vi "simplePID.vi"(8 "PID Gains":cluster{"Kp":dbl, "Kd":dbl, "Ki":dbl}, 10 "Position":dbl, 11 "Reference":dbl) -> (3 "control":dbl)   [LabVIEW 2010, in "kevLib2011.lvlib"]
uses:
  kevLib2011.lvlib
panel:
  # "Not Tested yet"
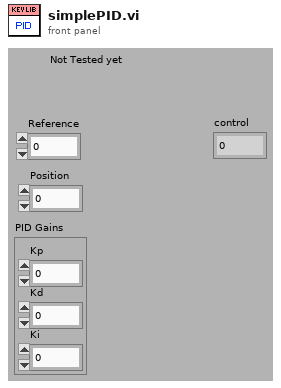
[diagram p1: front panel]
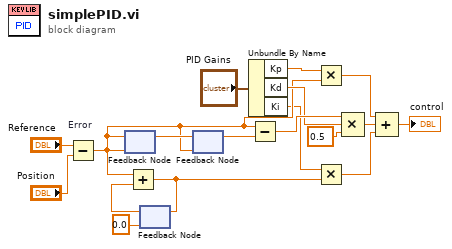
[diagram p0: block diagram]
diagram:
  n1 = Subtract "Error"(x="Reference", y="Position") -> (x-y=w7:dbl)
  n2 = feedback-in #1(w7) -> ()
  n3 = feedback #1(w7) -> (w13:dbl)
  n4 = feedback #2(0.0 ("value")) -> (w6:dbl)
  n5 = Add(x=w7, y=w6) -> (x+y=w3:dbl)
  n6 = feedback-in #2(w3) -> ()
  n7 = feedback-in #3(w13) -> ()
  n8 = feedback #3(w7) -> (w12:dbl)
  n9 = Unbundle By Name("PID Gains") -> ("Kp"=w15:dbl, "Kd"=w10:dbl, "Ki"=w4:dbl)
  n10 = Subtract(x=w7, y=w12) -> (x-y=w11:dbl)
  n11 = Multiply(x=w15, y=w7) -> (x*y=w14:dbl)
  n12 = Multiply(x=w4, y=w3) -> (x*y=w2:dbl)
  n13 = Compound Arithmetic op=MULTIPLY(w11, w10, 0.5 ("value")) -> (w8:dbl)
  n14 = Compound Arithmetic op=ADD(w14, w8, w2) -> (→"control":dbl)
